vi "CryoDC.vi"() -> ()   [LabVIEW 2017]
panel:
  in  "stop":bool
  out "Ch-15 2":sgl(slide) step=1 scale=-10.0..10.0 scale format="%.2f"
  out "Connected":bool
  out "bytes written":i32
  out "error out":errorcluster
  in  "remote port":u16=12345
  in  "address":string="192.168.1.203"
  in  "Depth":dbl(slide)=1.0 min=0.0 max=2.0 step=0.002 scale=0.0..2.0
  in  "clear":bool
  out "chd 15":dbl
  out "chd 14":dbl
  out "chd 13":dbl
  out "chd 12":dbl
  out "chd 11":dbl
  out "chd 10":dbl
  out "chd 9":dbl
  out "chd 8":dbl
  out "chd 7":dbl
  out "chd 6":dbl
  out "chd 5":dbl
  out "chd 4":dbl
  out "chd 3":dbl
  out "chd 2":dbl
  out "chd 1":dbl
  out "chd 0":dbl
  in  "ch 15":T1
  in  "ch 14":T1
  in  "ch 13":T1
  in  "ch 12":T1
  in  "ch 11":T1
  in  "ch 10":T1
  in  "ch 9":T1
  in  "ch 8":T1
  in  "ch 7":T1
  in  "ch 6":T1
  in  "ch 5":T1
  in  "ch 4":T1
  in  "ch 3":T1
  in  "ch 1":T1
  in  "ch 2":T1
  in  "ch 0":T1
  in  "Lateral":dbl(slide) min=-2.0 max=2.0 step=0.002 scale=-2.0..2.0
  in  "Vertical":dbl(slide) min=-2.0 max=2.0 step=0.001 scale=-2.0..2.0
  in  "Horizontal":dbl(slide) min=-2.0 max=2.0 step=0.002 scale=-2.0..2.0
  in  "Ch-15":sgl(slide) step=1 scale=-10.0..10.0 scale format="%.2f"
  in  "Ch-14":sgl(slide) step=1 scale=-10.0..10.0 scale format="%.2f"
  in  "Ch-13":sgl(slide) step=1 scale=-10.0..10.0 scale format="%.2f"
  in  "Ch-12":sgl(slide) step=1 scale=-10.0..10.0 scale format="%.2f"
  in  "Ch-11":sgl(slide) step=1 scale=-10.0..10.0 scale format="%.2f"
  in  "Ch-10":sgl(slide) step=1 scale=-10.0..10.0 scale format="%.2f"
  in  "Ch-9":sgl(slide) step=1 scale=-10.0..10.0 scale format="%.2f"
  in  "Ch-8":sgl(slide) step=1 scale=-10.0..10.0 scale format="%.2f"
  in  "Ch-7":sgl(slide) step=1 scale=-10.0..10.0 scale format="%.2f"
  in  "Ch-6":sgl(slide) step=1 scale=-10.0..10.0 scale format="%.2f"
  in  "Ch-5":sgl(slide) step=1 scale=-10.0..10.0 scale format="%.2f"
  in  "Ch-4":sgl(slide) step=1 scale=-10.0..10.0 scale format="%.2f"
  in  "Ch-2":sgl(slide) step=1 scale=-10.0..10.0 scale format="%.2f"
  in  "Ch-1":sgl(slide) step=1 scale=-10.0..10.0 scale format="%.2f"
  in  "Ch-3":sgl(slide) step=1 scale=-10.0..10.0 scale format="%.2f"
  in  "Ch-0":sgl(slide) step=1 scale=-10.0..10.0 scale format="%.2f"
  # "vertical"
  # "horizontal"
  # "+"
  # "lateral"
  # "+"
  # "A26"
  # "B7"
  # "B19"
  # "B2"
  # "B50"
  # "B28"
  # "PCI-6208V D/A Voltage Sample"
  # "B35"
  # "NC"
  # "B5"
  # "B33"
  # "NC"
  # "A39"
  # "A43"
  # "A27"
  # "A22"
  # "B30"
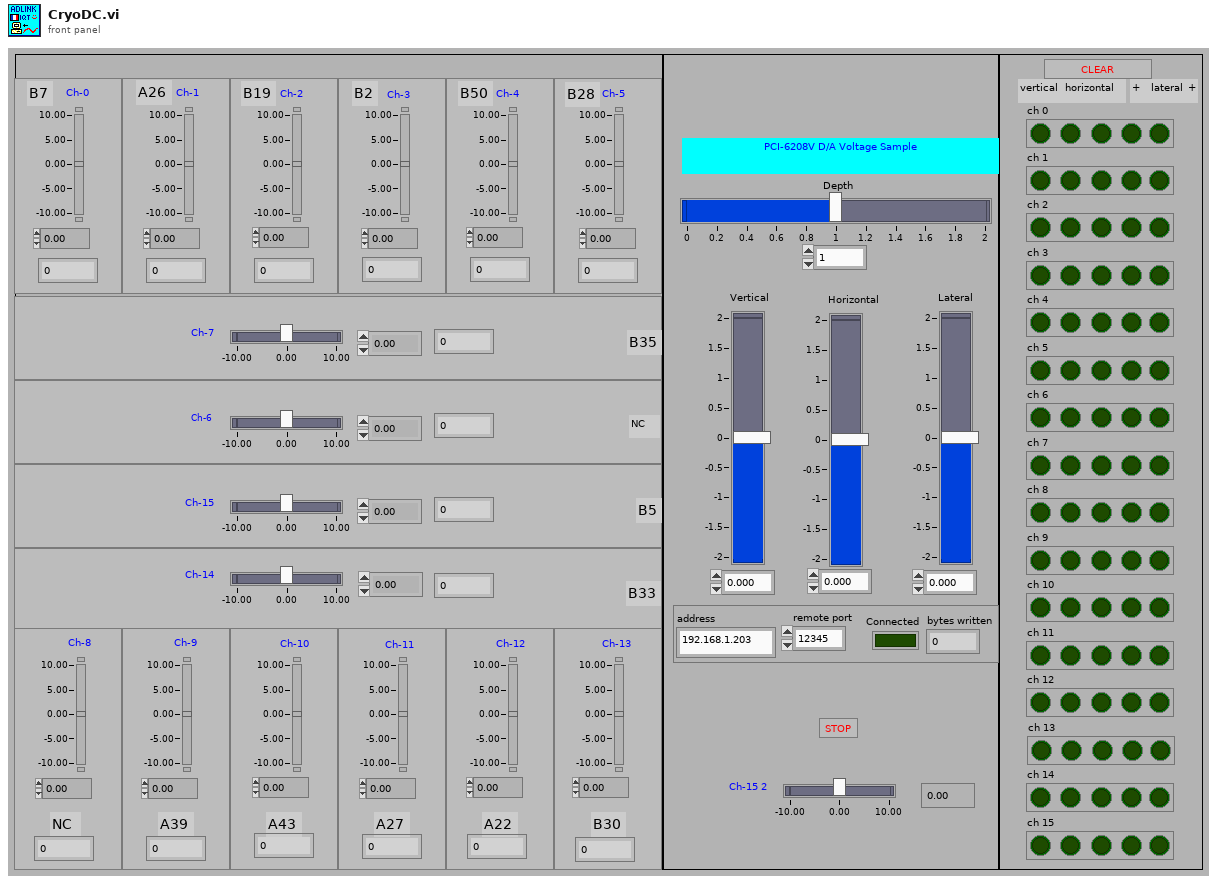
[diagram p1: front panel]
types:
  T1 = cluster{"vertical":bool, "horizontal":bool, "sign horizontal":bool, "lateral":bool, "sign lateral":bool}
  T2 = cluster{"vertical":bool, "horizontal":bool, "sign horizontal":bool, "lateral":bool, "sign lateral":bool}[]
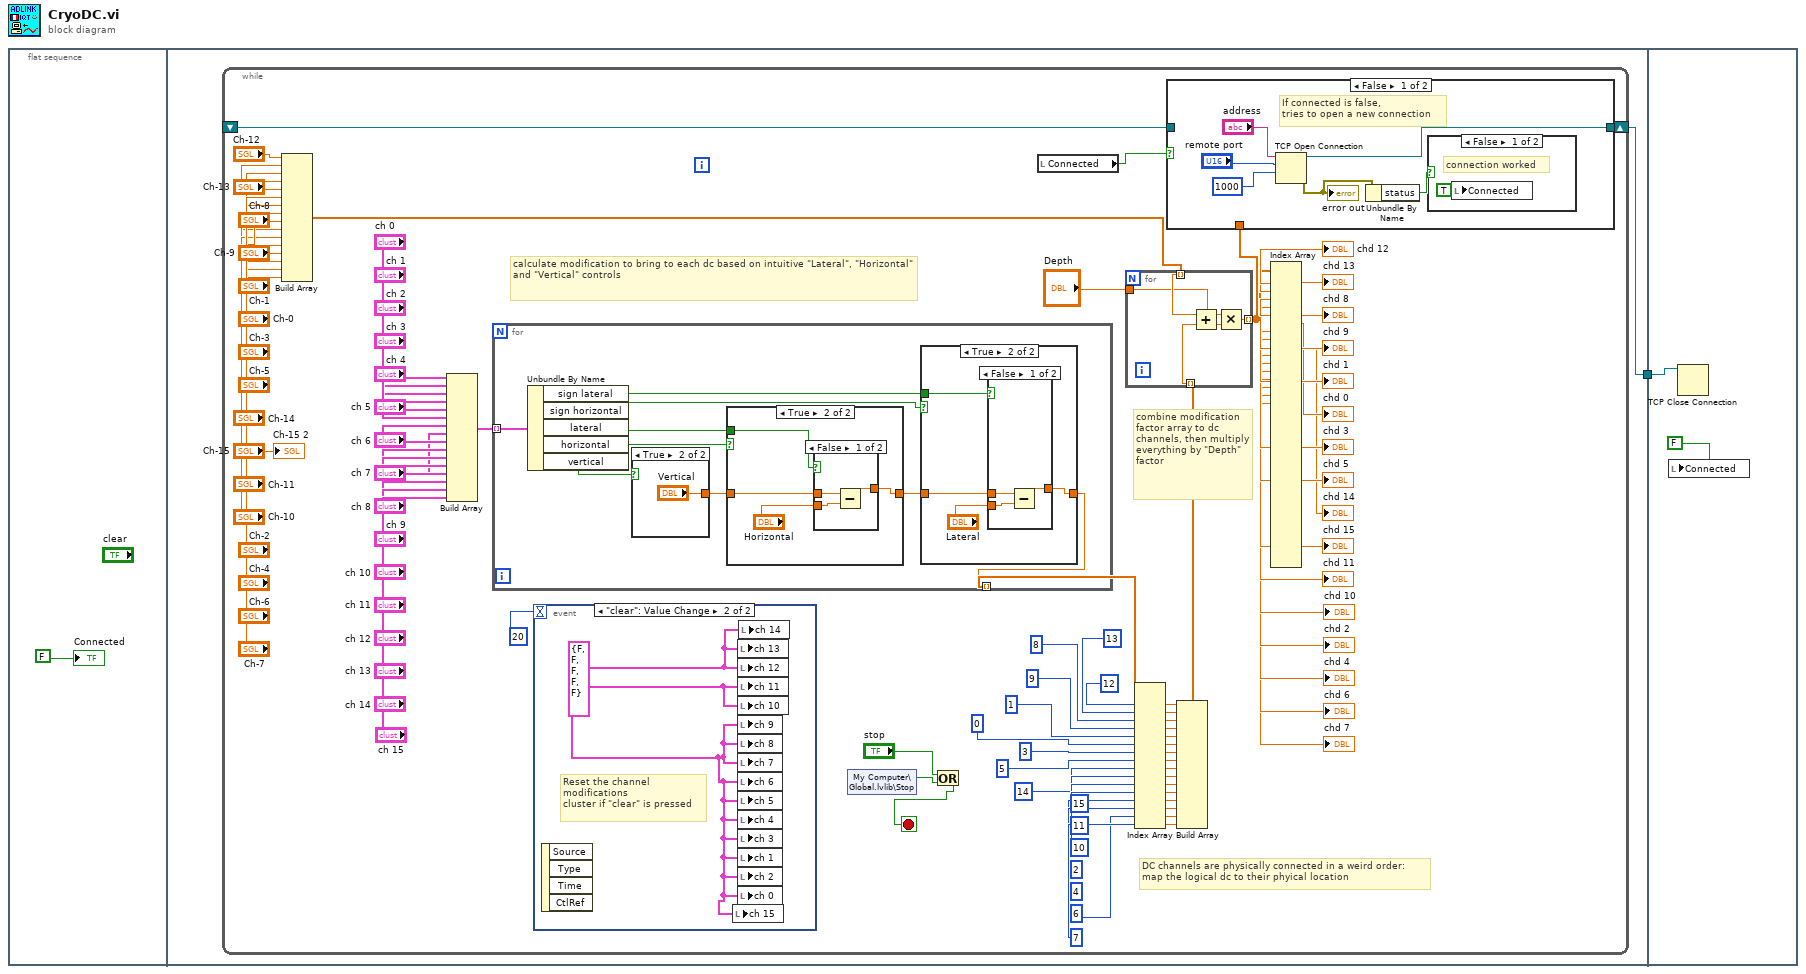
[diagram p0: block diagram]
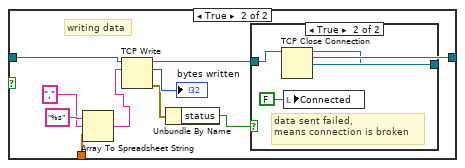
[diagram p3: hidden frame]
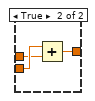
[diagram p6: hidden frame]
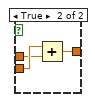
[diagram p8: hidden frame]
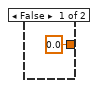
[diagram p9: hidden frame]
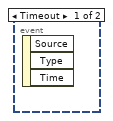
[diagram p10: hidden frame]
diagram:
  n1 = flat-sequence {
    tunnel: [w3] -> w1
    tunnel: w1 -> [w158]
    frame #0 {
      "Connected" <- FALSE ("Connected")
    }
    frame #1 {
      n2 = while {
        shift-right: [w9] -> w3
        shift-left: _ -> [w11]
        stop <- w4 stop-if-true
        # "calculate modification to bring to each dc based on intuitive \"Lateral\", \"Horizontal\" and \"Vertical\" controls"
        # "combine modification factor array to dc channels, then multiply everything by \"Depth\" factor"
        # "DC channels are physically connected in a weird order:\nmap the logical dc to their phyical location"
        n3 = Build Array("Ch-12", "Ch-13", "Ch-8", "Ch-9", "Ch-1", "Ch-0", "Ch-3", "Ch-5", "Ch-14", "Ch-15", "Ch-11", "Ch-10", "Ch-2", "Ch-4", "Ch-6", "Ch-7") -> (w30:sgl[])
        n4 = Build Array("ch 0", "ch 1", "ch 2", "ch 3", "ch 4", "ch 5", "ch 6", "ch 7", "ch 8", "ch 9", "ch 10", "ch 11", "ch 12", "ch 13", "ch 14", "ch 15") -> (w47:T2)
        n5 = for {
          tunnel: w47 -> [w131] mode=indexing
          tunnel: [w125] -> w48 mode=indexing
          n6 = Unbundle By Name(w131) -> ("sign lateral"=w123:bool, "sign horizontal"=w124:bool, "lateral"=w129:bool, "horizontal"=w130:bool, "vertical"=w128:bool)
          n7 = case shown="True" w128 {
            tunnel: [0.0 "Vertical"] -> w127
            frame False {
            }
            frame True {
            }
          }
          n8 = case shown="True" w130 {
            tunnel: w127 -> [w143 w145]
            tunnel: [w143 w144] -> w126
            tunnel: w124 -> [_ w147]
            frame False {
            }
            frame True {
              n9 = case shown="False" w147 {
                tunnel: "Horizontal" -> [w149 w153]
                tunnel: w145 -> [w150 w152]
                tunnel: [w148 w151] -> w144
                frame False {
                  n10 = Subtract(x=w150, y=w149) -> (x-y=w148:dbl)
                }
                frame True {
                  n11 = Add(x=w153, y=w152) -> (x+y=w151:dbl)
                }
              }
            }
          }
          n12 = case shown="True" w129 {
            tunnel: w126 -> [w132 w136]
            tunnel: [w132 w134] -> w125
            tunnel: w123 -> [_ w133]
            frame False {
            }
            frame True {
              n13 = case shown="False" w133 {
                tunnel: "Lateral" -> [w138 w142]
                tunnel: w136 -> [w139 w141]
                tunnel: [w137 w140] -> w134
                frame False {
                  n14 = Subtract(x=w139, y=w138) -> (x-y=w137:dbl)
                }
                frame True {
                  n15 = Add(x=w142, y=w141) -> (x+y=w140:dbl)
                }
              }
            }
          }
        }
        n16 = event shown="[1] \"clear\": Value Change" {
          selector: _ -> [_ _]
          dyn-events: _ -> [_ _]
          timeout: 20 -> [_ _]
          event Timeout {
            n17 = event-data() -> ()  [unwired: 1 in, 3 out]
          }
          event "clear": Value Change {
            w156 = T1 {"vertical"=FALSE, "horizontal"=FALSE, "sign horizontal"=FALSE, "lateral"=FALSE, "sign lateral"=FALSE} ("ch 15")
            # "Reset the channel modifications\ncluster if \"clear\" is pressed"
            n18 = event-data() -> ()  [unwired: 1 in, 4 out]
            n19 = local write "ch 15"(w156) -> ()
            n20 = local write "ch 13"(w156) -> ()
            n21 = local write "ch 12"(w156) -> ()
            n22 = local write "ch 11"(w156) -> ()
            n23 = local write "ch 10"(w156) -> ()
            n24 = local write "ch 9"(w156) -> ()
            n25 = local write "ch 8"(w156) -> ()
            n26 = local write "ch 7"(w156) -> ()
            n27 = local write "ch 6"(w156) -> ()
            n28 = local write "ch 5"(w156) -> ()
            n29 = local write "ch 4"(w156) -> ()
            n30 = local write "ch 3"(w156) -> ()
            n31 = local write "ch 1"(w156) -> ()
            n32 = local write "ch 2"(w156) -> ()
            n33 = local write "ch 0"(w156) -> ()
            n34 = local write "ch 14"(w156) -> ()
          }
        }
        n35 = shared-variable "My Computer\\Global.lvlib\\Stop"() -> (w6:bool)  [unwired: 1 in, 1 out]
        n36 = Or(x="stop", y=w6) -> (x .or. y?=w4:bool)
        n37 = local read "Connected"() -> (w8:bool)
        n38 = Index Array(array=w48, index #1=12 ("index"), index #2=13 ("index"), index #3=8 ("index"), index #4=9 ("index"), index #5=1 ("index"), index #6=0 ("index"), index #7=3 ("index"), index #8=5 ("index"), index #9=14 ("index"), index #10=15 ("index"), index #11=11 ("index"), index #12=10 ("index"), index #13=2 ("index"), index #14=4 ("index"), index #15=6 ("index"), index #16=7 ("index")) -> (element #1=w51:dbl, element #2=w52:dbl, element #3=w66:dbl, element #4=w67:dbl, element #5=w68:dbl, element #6=w69:dbl, element #7=w70:dbl, element #8=w71:dbl, element #9=w72:dbl, element #10=w73:dbl, element #11=w74:dbl, element #12=w75:dbl, element #13=w76:dbl, element #14=w77:dbl, element #15=w78:dbl, element #16=w79:dbl)
        n39 = Build Array(w51, w52, w66, w67, w68, w69, w70, w71, w72, w73, w74, w75, w76, w77, w78, w79) -> (w29:dbl[])
        n40 = for {
          tunnel: w30 -> [w122] mode=indexing
          tunnel: w29 -> [w121] mode=indexing
          tunnel: [w119] -> w10 mode=indexing
          tunnel: "Depth" -> [w118]
          n41 = Add(x=w122, y=w121) -> (x+y=w120:dbl)
          n42 = Multiply(x=w118, y=w120) -> (x*y=w119:dbl)
        }
        n43 = case shown="False" w8 {
          tunnel: w11 -> [_ w113]
          tunnel: w10 -> [_ w110]
          tunnel: [w100 w104] -> w9
          frame False {
            # "If connected is false,\ntries to open a new connection"
            n44 = TCP Open Connection(address="address", remote port or service name="remote port", timeout ms (60000)=1000) -> (connection ID=w100:refnum<k5>, error out=w98:errorcluster)  [unwired: 2 in]
            "error out" <- w98
            n45 = Unbundle By Name(w98) -> ("status"=w97:bool)
            n46 = case shown="False" w97 {
              frame False {
                # "connection worked"
                n47 = local write "Connected"(TRUE ("Connected")) -> ()
              }
              frame True {
              }
            }
          }
          frame True {
            # "writing data"
            n48 = Array To Spreadsheet String(delimiter (Tab)=",", array=w110, 3:"%s" ("format string")) -> (spreadsheet string=w108:string)
            n49 = TCP Write(connection ID=w113, data in=w108) -> (connection ID out=w105:refnum<k5>, bytes written=→"bytes written":i32, error out=w107:errorcluster)  [unwired: 2 in]
            n50 = Unbundle By Name(w107) -> ("status"=w106:bool)
            n51 = case shown="True" w106 {
              tunnel: w105 -> [w114 w116]
              tunnel: [w114 w115] -> w104
              frame False {
              }
              frame True {
                # "data sent failed,\nmeans connection is broken"
                n52 = TCP Close Connection(connection ID=w116) -> (connection ID out=w115:refnum<k5>)  [unwired: 2 in, 1 out]
                n53 = local write "Connected"(FALSE ("Connected")) -> ()
              }
            }
          }
        }
        n54 = Index Array(array=w10) -> (element #1=→"chd 12":dbl, element #2=→"chd 13":dbl, element #3=→"chd 8":dbl, element #4=→"chd 9":dbl, element #5=→"chd 1":dbl, element #6=→"chd 0":dbl, element #7=→"chd 3":dbl, element #8=→"chd 5":dbl, element #9=→"chd 14":dbl, element #10=→"chd 15":dbl, element #11=→"chd 11":dbl, element #12=→"chd 10":dbl, element #13=→"chd 2":dbl, element #14=→"chd 4":dbl, element #15=→"chd 6":dbl, element #16=→"chd 7":dbl)  [unwired: 36 in, 20 out]
        "Ch-15 2" <- "Ch-15"
      }
    }
    frame #2 {
      n55 = local write "Connected"(FALSE) -> ()
      n56 = TCP Close Connection(connection ID=w158) -> ()  [unwired: 2 in, 2 out]
    }
  }
